vi "Make Channels Coincident.vi"(6 "interp. method":i32(ring) items=["nearest", "linear", "spline", "cubic Hermite", "Lagrange"], 8 "Time Cluster 2":T1, 9 "Time Cluster 1":T1, 10 "Cluster 2":T2={"Colour"=0, "Inst type"=enum."Pitot-static tube", "Inst name"="Manometer voltage", "Symbol"="U", "Code name"="", "Extra Info"="U", "Inst Array"=enum."PWA", "Extra Titles"=[], "Extra Values"=[], "U"=0.0, "u^2"=0.0, "u^3"=0.0, "u^4"=0.0, "Skew_u"=0.0, "Kurt_u"=0.0, "Sd Error in Mean"=0.0, "% u'/U"=0.0, "X"=0.0, "Y"=0.0, "Z"=0.0, "Timescale integral Estimate"=0.0, "Sd Error in Variance"=0.0, "Calib File"=path "", "Calib Constants"=[], "Output Position"=FALSE, "Full Stats"=FALSE, "Av Sampling Rate"=0.0, "Av No of Samples"=0.0, "Total Meas Time (s)"=0.0, "ADAM Ch Name"="", "Max value"=0.0, "Min value"=0.0, "Sync Delay Time (s)"=0.0} {"Sync Delay Time (s)" format="%.2f"; "Sd Error in Variance" format="%.2f"; "Skew_u" format="%.2f"; "% u'/U" format="%.2f"; "Sd Error in Mean" format="%.2f"; "Kurt_u" format="%.2f"; "u^4" format="%.2f"; "u^3" format="%.2f"; "U" format="%.2f"; "u^2" format="%.2f"}, 11 "Cluster 1":T2={"Colour"=0, "Inst type"=enum."Pitot-static tube", "Inst name"="Manometer voltage", "Symbol"="U", "Code name"="", "Extra Info"="U", "Inst Array"=enum."PWA", "Extra Titles"=[], "Extra Values"=[], "U"=0.0, "u^2"=0.0, "u^3"=0.0, "u^4"=0.0, "Skew_u"=0.0, "Kurt_u"=0.0, "Sd Error in Mean"=0.0, "% u'/U"=0.0, "X"=0.0, "Y"=0.0, "Z"=0.0, "Timescale integral Estimate"=0.0, "Sd Error in Variance"=0.0, "Calib File"=path "", "Calib Constants"=[], "Output Position"=FALSE, "Full Stats"=FALSE, "Av Sampling Rate"=0.0, "Av No of Samples"=0.0, "Total Meas Time (s)"=0.0, "ADAM Ch Name"="", "Max value"=0.0, "Min value"=0.0, "Sync Delay Time (s)"=0.0} {"Sync Delay Time (s)" format="%.2f"; "Sd Error in Variance" format="%.2f"; "Skew_u" format="%.2f"; "% u'/U" format="%.2f"; "Sd Error in Mean" format="%.2f"; "Kurt_u" format="%.2f"; "u^4" format="%.2f"; "u^3" format="%.2f"; "U" format="%.2f"; "u^2" format="%.2f"}) -> (1 "Coincident Time Cluster 2":T1, 3 "Coincident Time Cluster 1":T1)   [LabVIEW 2017]
uses:
  Controls/Analysis_info_cluster.ctl
  Controls/Inst_type.ctl
  Controls/Instrument_Array.ctl
  Controls/Time_Trace_Cluster.ctl
  <vilib>/gmath/NI_Gmath.lvlib
panel:
  out "Time (s)":dbl[](array[numeric])
  in  "Show Plots":bool
  out "U1 and U2 Raw":cluster{"yi":dbl[], "yi":dbl[]}[](graph)
  out "U1 and U2 made coincident":cluster{"yi":dbl[], "yi":dbl[]}[](graph)
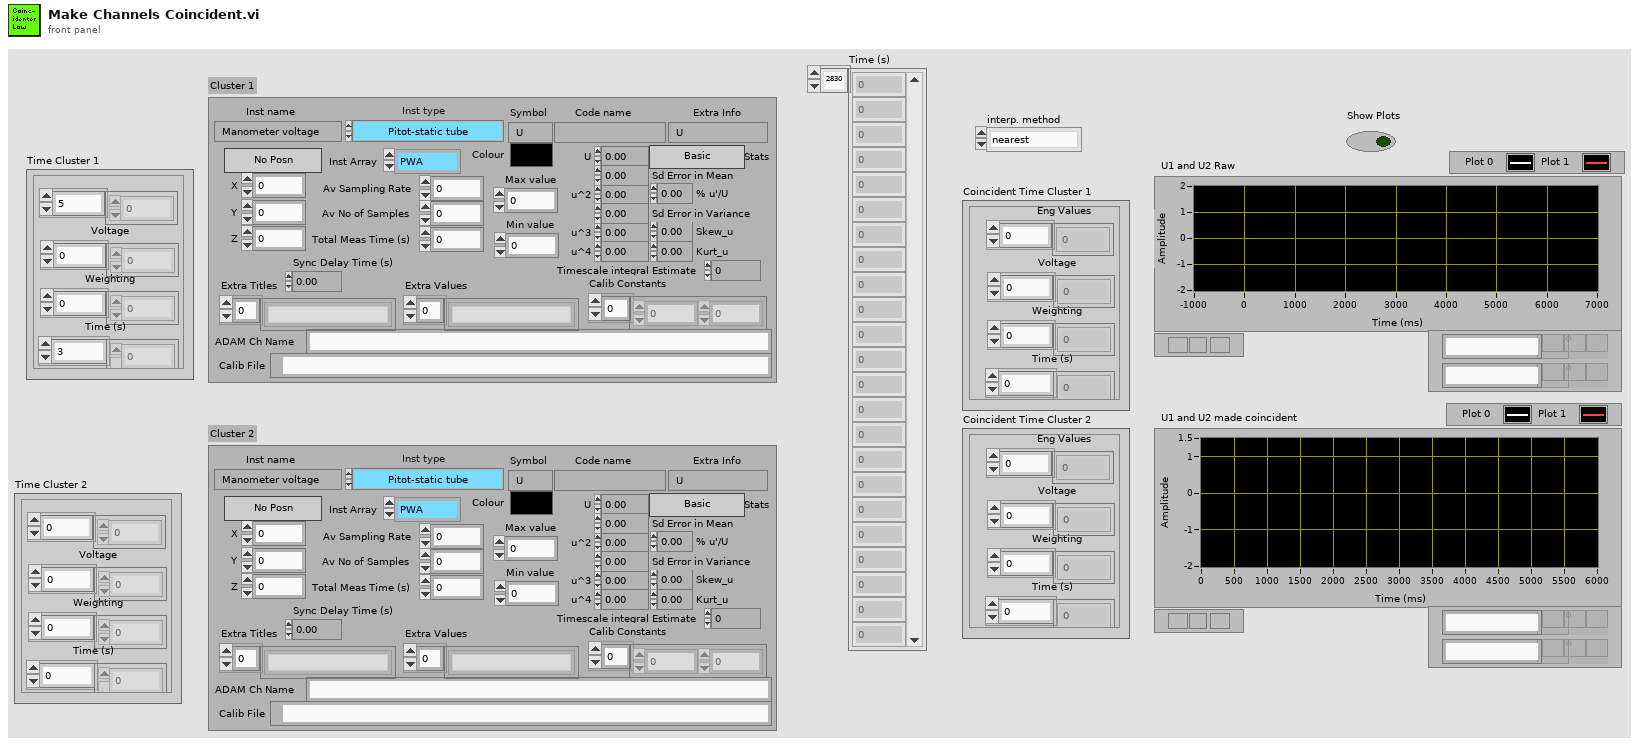
[diagram p1: front panel]
types:
  T1 = typedef "Time_Trace_Cluster.ctl" = cluster{"Weighting":dbl[], "Time (s)":dbl[], "Voltage":dbl[], "Eng Values":dbl[]}
  T2 = typedef "Analysis_info_cluster.ctl" = cluster{"Colour":u32, "Inst type":T3, "Inst name":string, "Symbol":string, "Code name":string, "Extra Info":string, "Inst Array":T4, "Extra Titles":string[], "Extra Values":string[], "U":dbl, "u^2":dbl, "u^3":dbl, "u^4":dbl, "Skew_u":dbl, "Kurt_u":dbl, "Sd Error in Mean":dbl, "% u'/U":dbl, "X":dbl, "Y":dbl, "Z":dbl, "Timescale integral Estimate":dbl, "Sd Error in Variance":dbl, "Calib File":path, "Calib Constants":dbl[], "Output Position":bool, "Full Stats":bool, "Av Sampling Rate":dbl, "Av No of Samples":dbl, "Total Meas Time (s)":dbl, "ADAM Ch Name":string, "Max value":dbl, "Min value":dbl, "Sync Delay Time (s)":dbl}
  T3 = typedef "Inst_type.ctl" = enum16{"Propeller anemometer", "Raw voltage", "Pressure Transducer", "Pitot-static tube", "Preston tube", "Hot wire", "Cross wire 1", "Cross wire 2", "Generic Linear", "Generic Polynomial", "Generic BackPoly", "Fast FID", "Thermocouple", "Cold wire", "Pulsed Wire", "LDA Vel", "LDA Tran time", "LDA Arr time", "Microphone"}
  T4 = typedef "Instrument_Array.ctl" = enum16{"PWA", "LDA", "Analogue"}
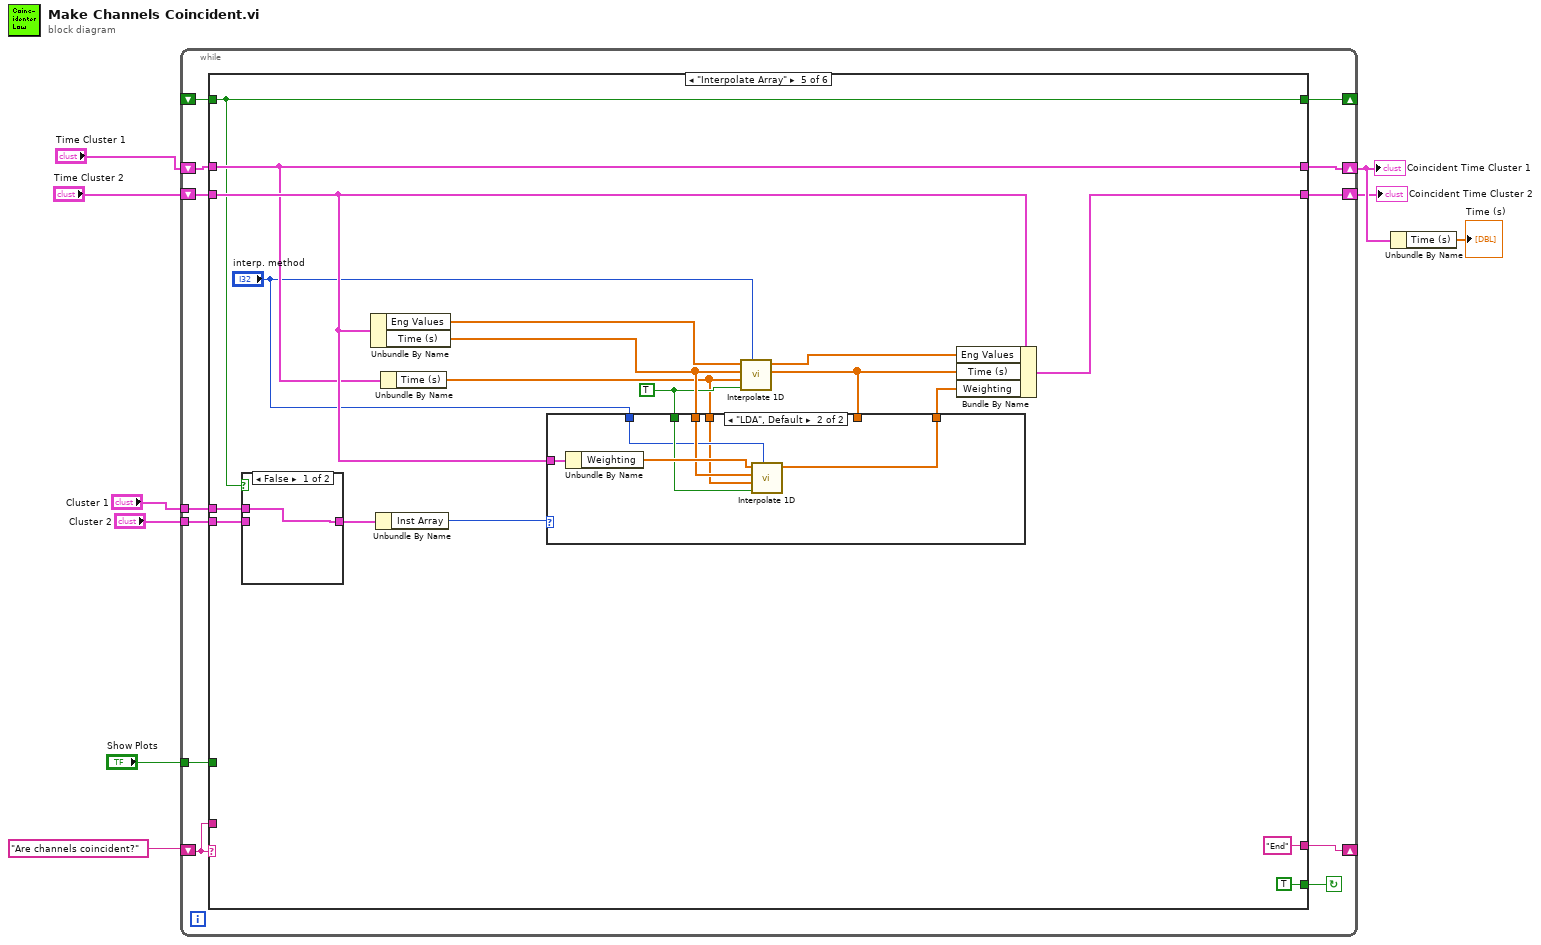
[diagram p0: block diagram]
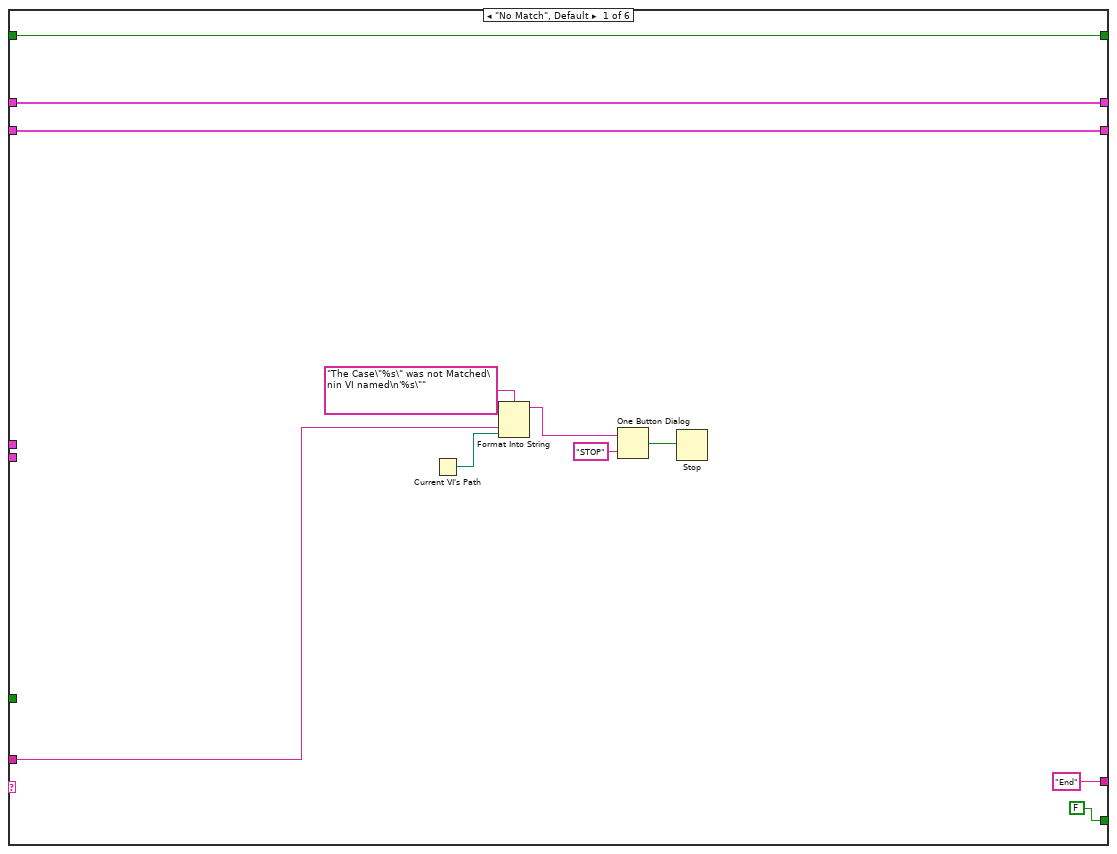
[diagram p2: hidden frame]
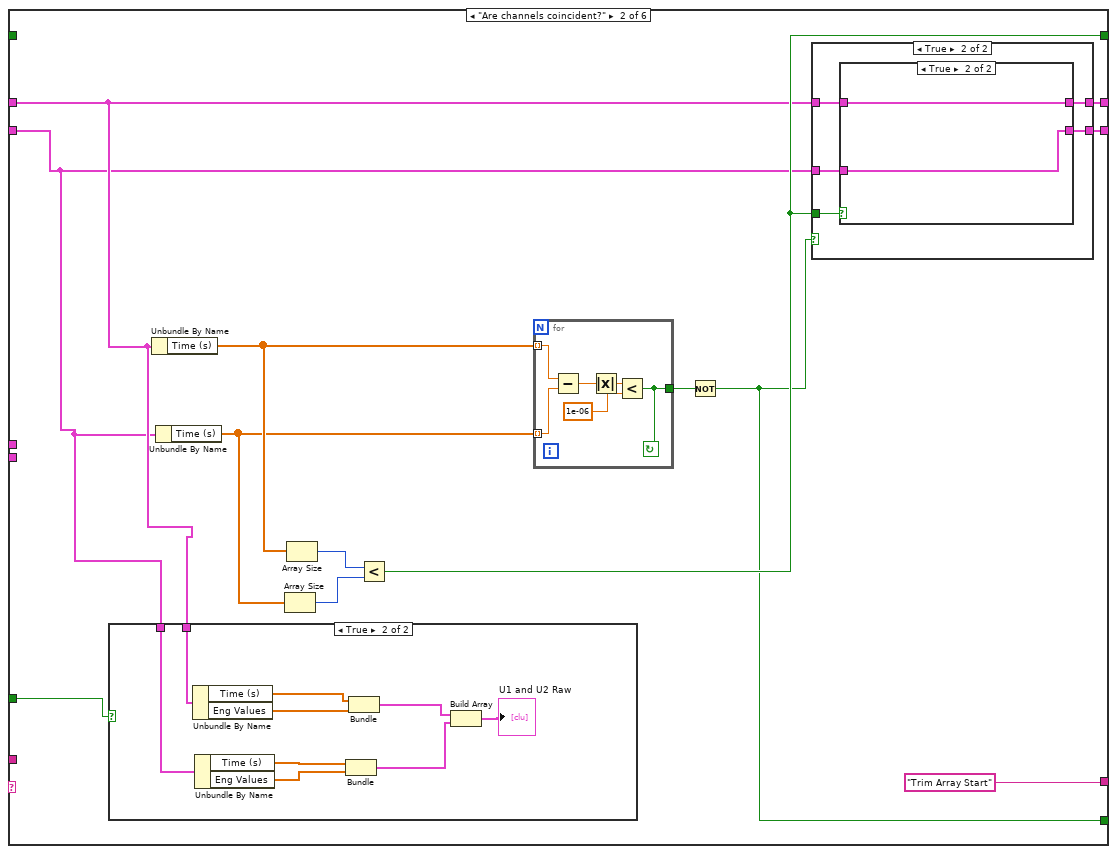
[diagram p3: hidden frame]
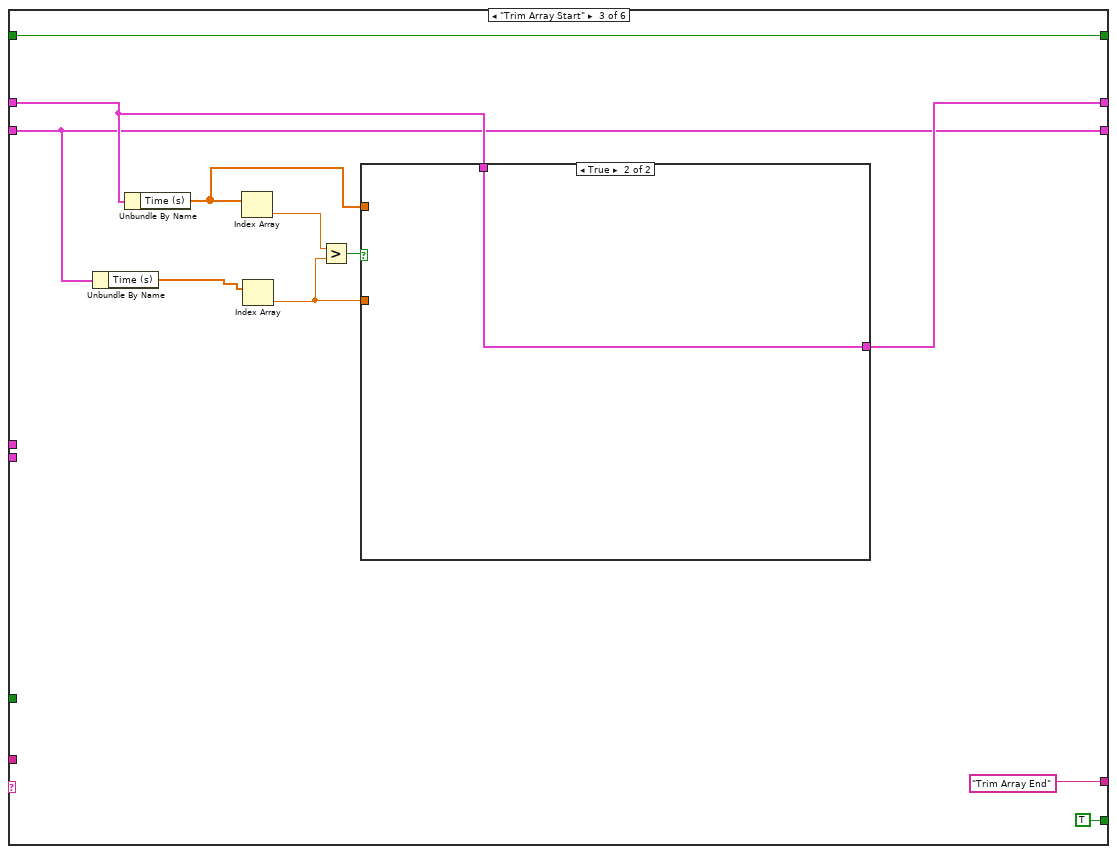
[diagram p7: hidden frame]
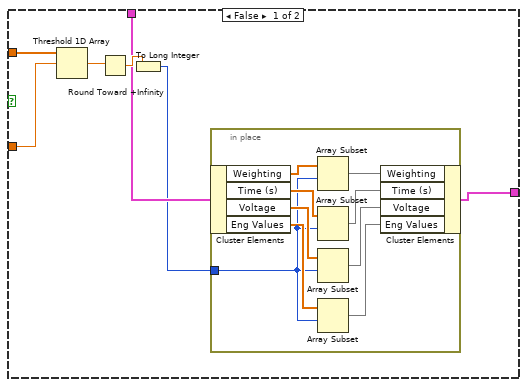
[diagram p8: hidden frame]
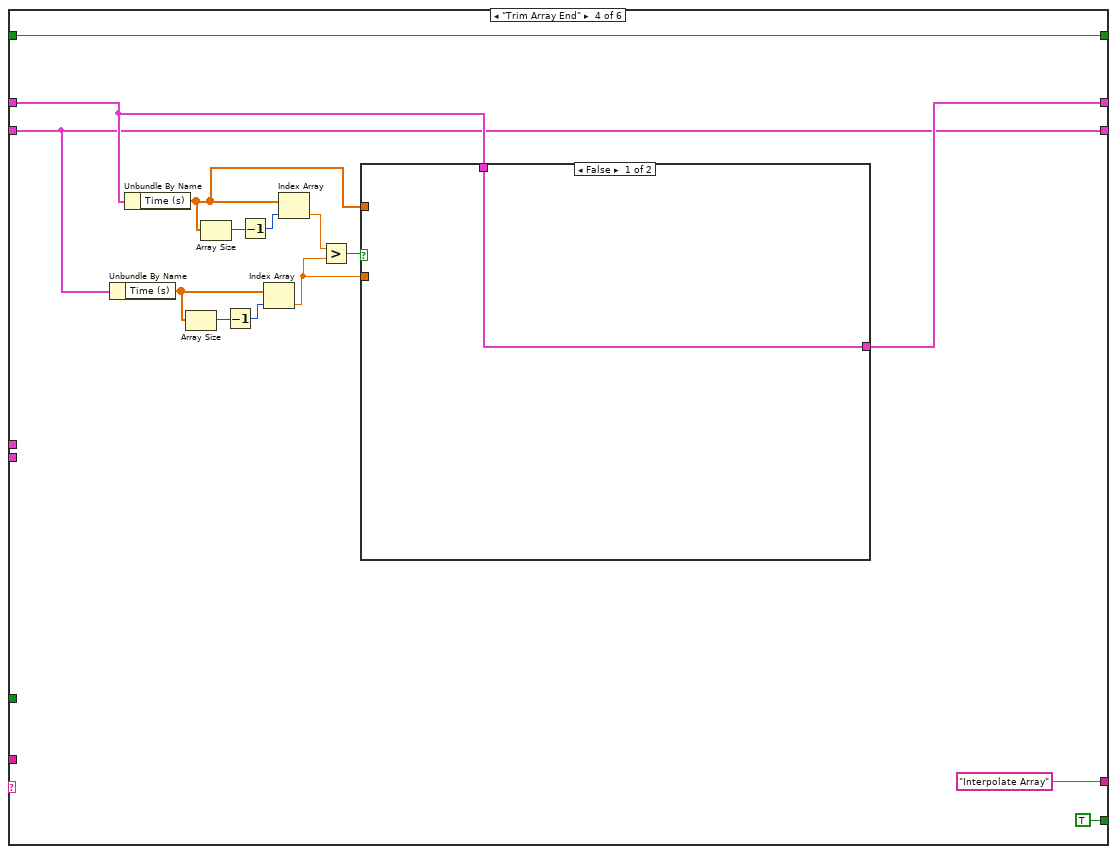
[diagram p9: hidden frame]
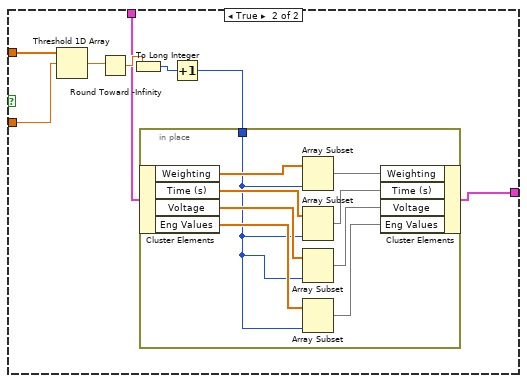
[diagram p10: hidden frame]
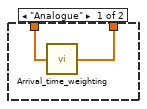
[diagram p12: hidden frame]
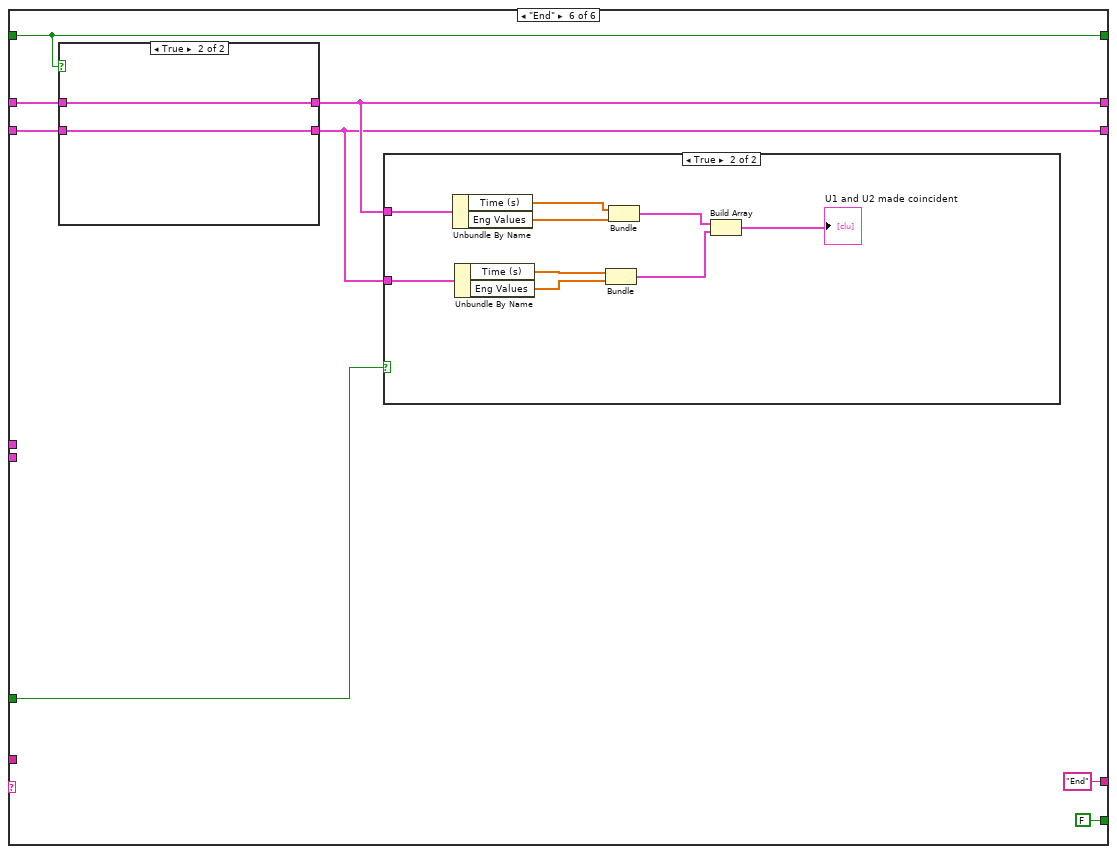
[diagram p13: hidden frame]
diagram:
  n1 = while {
    shift-right: [w16] -> w3
    shift-left: "Time Cluster 1" -> [w18]
    shift-right: [w15] -> w2
    shift-left: "Time Cluster 2" -> [w17]
    shift-right: [w19] -> _
    shift-left: "Are channels coincident?" -> [w21]
    tunnel: "Show Plots" -> [w14]
    tunnel: "Cluster 1" -> [w13]
    tunnel: "Cluster 2" -> [w12]
    shift-right: [w11] -> _
    shift-left: _ -> [w10]
    stop <- w20 continue-if-true
    n2 = case shown="\"Interpolate Array\"" w21 {
      tunnel: w21 -> [w27 _ _ _ _ _]
      tunnel: [FALSE w33 TRUE TRUE TRUE FALSE] -> w20
      tunnel: ["End" "Trim Array Start" "Trim Array End" "Interpolate Array" ("t") "End" "End" ("t")] -> w19
      tunnel: w18 -> [w24 w35 w79 w111 w140 w165]
      tunnel: w17 -> [w23 w34 w78 w103 w142 w163]
      tunnel: [w24 w38 w80 w112 w140 w166] -> w16
      tunnel: [w23 w39 w78 w103 w141 w164] -> w15
      tunnel: w14 -> [_ w36 _ _ _ w167]
      tunnel: w13 -> [_ _ _ _ w133 _]
      tunnel: w12 -> [_ _ _ _ w134 _]
      tunnel: [w22 w37 w73 w101 w136 w162] -> w11
      tunnel: w10 -> [w22 _ w73 w101 w136 w162]
      frame "No Match", Default {
        n3 = Current VI's Path() -> (path=w32:path)
        n4 = Format Into String(format string="The Case\"%s\" was not Matched\nin VI named\n'%s\"" ("Format String"), w27, w32) -> (resulting string=w29:string)  [unwired: 2 in, 1 out]
        n5 = One Button Dialog(message=w29, button name ("OK")="STOP") -> (true=w31:bool)
        n6 = Stop(stop? (T)=w31) -> ()
      }
      frame "Are channels coincident?" {
        n7 = case shown="True" w36 {
          tunnel: w35 -> [_ w58]
          tunnel: w34 -> [_ w57]
          frame False {
          }
          frame True {
            n8 = Unbundle By Name(w58) -> ("Time (s)"=w59:dbl[], "Eng Values"=w63:dbl[])
            n9 = Unbundle By Name(w57) -> ("Time (s)"=w60:dbl[], "Eng Values"=w62:dbl[])
            n10 = Bundle("Time (s)"=w60, "Eng Values"=w62) -> (w61:cluster{"Time (s)":dbl[], "Eng Values":dbl[]})  [unwired: 1 in]
            n11 = Bundle("Time (s)"=w59, "Eng Values"=w63) -> (w64:cluster{"Time (s)":dbl[], "Eng Values":dbl[]})  [unwired: 1 in]
            n12 = Build Array(w64, w61) -> (→"U1 and U2 Raw":cluster{"Time (s)":dbl[], "Eng Values":dbl[]}[])
          }
        }
        n13 = Unbundle By Name(w35) -> ("Time (s)"=w41:dbl[])
        n14 = Unbundle By Name(w34) -> ("Time (s)"=w40:dbl[])
        n15 = Array Size(array=w40) -> (size(s)=w42:i32)
        n16 = Array Size(array=w41) -> (size(s)=w43:i32)
        n17 = Less?(x=w43, y=w42) -> (x < y?=w37:bool)
        n18 = for {
          tunnel: w41 -> [w68] mode=indexing
          tunnel: w40 -> [w67] mode=indexing
          tunnel: [w66] -> w44
          stop <- w66 continue-if-true
          n19 = Subtract(x=w68, y=w67) -> (x-y=w71:dbl)
          n20 = Absolute Value(x=w71) -> (abs(x)=w70:dbl)
          n21 = Less?(x=w70, y=1e-06) -> (x < y?=w66:bool)
        }
        n22 = Not(x=w44) -> (.not. x?=w33:bool)
        n23 = case shown="True" w33 {
          tunnel: [w46 w52] -> w39
          tunnel: [w47 w51] -> w38
          tunnel: w37 -> [_ w50]
          tunnel: w35 -> [w47 w49]
          tunnel: w34 -> [w46 w48]
          frame False {
          }
          frame True {
            n24 = case shown="True" w50 {
              tunnel: [w54 w55] -> w52
              tunnel: w49 -> [w54 w56]
              tunnel: w48 -> [w53 w55]
              tunnel: [w53 w56] -> w51
              frame False {
              }
              frame True {
              }
            }
          }
        }
      }
      frame "Trim Array Start" {
        n25 = Unbundle By Name(w78) -> ("Time (s)"=w75:dbl[])
        n26 = Unbundle By Name(w79) -> ("Time (s)"=w77:dbl[])
        n27 = Index Array(array=w77) -> (element=w76:dbl)  [unwired: 1 in]
        n28 = Index Array(array=w75) -> (element=w74:dbl)  [unwired: 1 in]
        n29 = Greater?(x=w76, y=w74) -> (0:w81:bool)
        n30 = case shown="True" w81 {
          tunnel: w77 -> [w89 _]
          tunnel: w74 -> [w88 _]
          tunnel: w79 -> [w85 w99]
          tunnel: [w83 w99] -> w80
          frame False {
            n31 = Threshold 1D Array(2:w88, 3:w89) -> (0:w87:dbl)  [unwired: 1 in]
            n32 = Round Toward +Infinity(x=w87) -> (ceil(x): smallest int >= x=w86:dbl)
            n33 = To Long Integer(number=w86) -> (32bit integer=w84:i32)
            n34 = in-place {
              in-place-border: w84 -> [w94]
              n35 = in-place-cluster #1(w85) -> ("Weighting"=w98:dbl[], "Time (s)"=w97:dbl[], "Voltage"=w96:dbl[], "Eng Values"=w95:dbl[])
              n36 = Array Subset(array=w98, index=w94) -> (w90:dbl[])  [unwired: 1 in]
              n37 = Array Subset(array=w97, index=w94) -> (w91:dbl[])  [unwired: 1 in]
              n38 = Array Subset(array=w96, index=w94) -> (w92:dbl[])  [unwired: 1 in]
              n39 = Array Subset(array=w95, index=w94) -> (w93:dbl[])  [unwired: 1 in]
              n40 = in-place-cluster #1("Weighting"=w90, "Time (s)"=w91, "Voltage"=w92, "Eng Values"=w93) -> (w83:T1)
            }
          }
          frame True {
          }
        }
      }
      frame "Trim Array End" {
        n41 = Unbundle By Name(w103) -> ("Time (s)"=w106:dbl[])
        n42 = Unbundle By Name(w111) -> ("Time (s)"=w109:dbl[])
        n43 = Array Size(array=w106) -> (size(s)=w105:i32)
        n44 = Array Size(array=w109) -> (size(s)=w108:i32)
        n45 = Decrement(x=w105) -> (x-1=w104:i32)
        n46 = Decrement(x=w108) -> (x-1=w107:i32)
        n47 = Index Array(array=w106, index=w104) -> (element=w102:dbl)
        n48 = Index Array(array=w109, index=w107) -> (element=w110:dbl)
        n49 = Greater?(x=w110, y=w102) -> (0:w113:bool)
        n50 = case shown="False" w113 {
          tunnel: w109 -> [_ w123]
          tunnel: w111 -> [w115 w120]
          tunnel: [w115 w119] -> w112
          tunnel: w102 -> [_ w118]
          frame False {
          }
          frame True {
            n51 = Threshold 1D Array(2:w118, 3:w123) -> (0:w122:dbl)  [unwired: 1 in]
            n52 = Round Toward -Infinity(1:w122) -> (0:w121:dbl)
            n53 = To Long Integer(number=w121) -> (32bit integer=w117:i32)
            n54 = Increment(x=w117) -> (x+1=w116:i32)
            n55 = in-place {
              in-place-border: w116 -> [w124]
              n56 = in-place-cluster #2(w120) -> ("Weighting"=w132:dbl[], "Time (s)"=w131:dbl[], "Voltage"=w130:dbl[], "Eng Values"=w129:dbl[])
              n57 = Array Subset(array=w132, length=w124) -> (w125:dbl[])  [unwired: 1 in]
              n58 = Array Subset(array=w131, length=w124) -> (w126:dbl[])  [unwired: 1 in]
              n59 = Array Subset(array=w130, length=w124) -> (w127:dbl[])  [unwired: 1 in]
              n60 = Array Subset(array=w129, length=w124) -> (w128:dbl[])  [unwired: 1 in]
              n61 = in-place-cluster #2("Weighting"=w125, "Time (s)"=w126, "Voltage"=w127, "Eng Values"=w128) -> (w119:T1)
            }
          }
        }
      }
      frame "Interpolate Array" {
        w147 = TRUE ("X is monotonic")
        n62 = case shown="False" w136 {
          tunnel: [w151 w152] -> w135
          tunnel: w134 -> [_ w152]
          tunnel: w133 -> [w151 _]
          frame False {
          }
          frame True {
          }
        }
        n63 = Unbundle By Name(w142) -> ("Eng Values"=w150:dbl[], "Time (s)"=w148:dbl[])
        n64 = Unbundle By Name(w135) -> ("Inst Array"=w139:T4)
        n65 = Unbundle By Name(w140) -> ("Time (s)"=w146:dbl[])
        n66 = call <vilib>:"Interpolate 1D.vi"("method"="interp. method", "X is monotonic"=w147, "xi"=w146, "X"=w148, "Y"=w150) -> ("xi used"=w144:dbl[], "yi"=w149:dbl[])  [unwired: 1 in, 4 out]
        n67 = case shown="\"LDA\", Default" w139 {
          tunnel: w142 -> [_ w159]
          tunnel: w148 -> [_ w160]
          tunnel: w147 -> [_ w158]
          tunnel: "interp. method" -> [_ w157]
          tunnel: w146 -> [_ w156]
          tunnel: [w153 w155] -> w145
          tunnel: w144 -> [w154 _]
          frame "Analogue" {
            n68 = call "Arrival_time_weighting.vi"("Arrival times"=w154) -> ("Weighting"=w153:dbl[])
          }
          frame "LDA", Default {
            n69 = Unbundle By Name(w159) -> ("Weighting"=w161:dbl[])
            n70 = call <vilib>:"Interpolate 1D.vi"("method"=w157, "X is monotonic"=w158, "xi"=w156, "X"=w160, "Y"=w161) -> ("yi"=w155:dbl[])  [unwired: 1 in, 5 out]
          }
        }
        n71 = Bundle By Name(cluster=w142, "Eng Values"=w149, "Time (s)"=w144, "Weighting"=w145) -> (w141:T1)
      }
      frame "End" {
        n72 = case shown="True" w162 {
          tunnel: [w170 w173] -> w166
          tunnel: w165 -> [w171 w173]
          tunnel: [w171 w172] -> w164
          tunnel: w163 -> [w170 w172]
          frame False {
          }
          frame True {
          }
        }
        n73 = case shown="True" w167 {
          tunnel: w166 -> [_ w182]
          tunnel: w164 -> [_ w181]
          frame False {
          }
          frame True {
            n74 = Unbundle By Name(w182) -> ("Time (s)"=w175:dbl[], "Eng Values"=w179:dbl[])
            n75 = Unbundle By Name(w181) -> ("Time (s)"=w176:dbl[], "Eng Values"=w178:dbl[])
            n76 = Bundle("Time (s)"=w176, "Eng Values"=w178) -> (w177:cluster{"Time (s)":dbl[], "Eng Values":dbl[]})  [unwired: 1 in]
            n77 = Bundle("Time (s)"=w175, "Eng Values"=w179) -> (w180:cluster{"Time (s)":dbl[], "Eng Values":dbl[]})  [unwired: 1 in]
            n78 = Build Array(w180, w177) -> (→"U1 and U2 made coincident":cluster{"Time (s)":dbl[], "Eng Values":dbl[]}[])
          }
        }
      }
    }
  }
  "Coincident Time Cluster 1" <- w3
  "Coincident Time Cluster 2" <- w2
  n79 = Unbundle By Name(w3) -> ("Time (s)"=→"Time (s)":dbl[])
